vi "Mapping Channel and Image.vi"(9 "Channel Info Index In":u16, 10 "Channel Name":string, 11 "Operation":T2(ring)) -> (1 "Channel Info Index Out":u16, 2 "Channel Info":T1)   [LabVIEW 2021, in "myRIOMetaDataObj.lvclass"]
uses:
  myRIOMetaDataObj.lvclass
  ChannelInfo.ctl
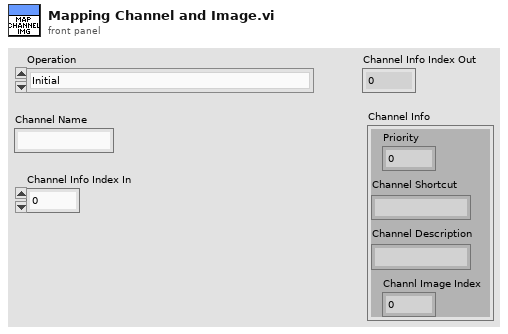
[diagram p1: front panel]
types:
  T1 = typedef "myRIOMetaDataObj.lvclass/ChannelInfo.ctl" = cluster{"Priority":u16, "Channel Shortcut":string, "Channel Description":string, "Channl Image Index":u16}
  T2 = enum16{"Initial", "Get Channel Info Index by Name", "Get Channel Info by Index", "Get Channel Info by Img Index"}
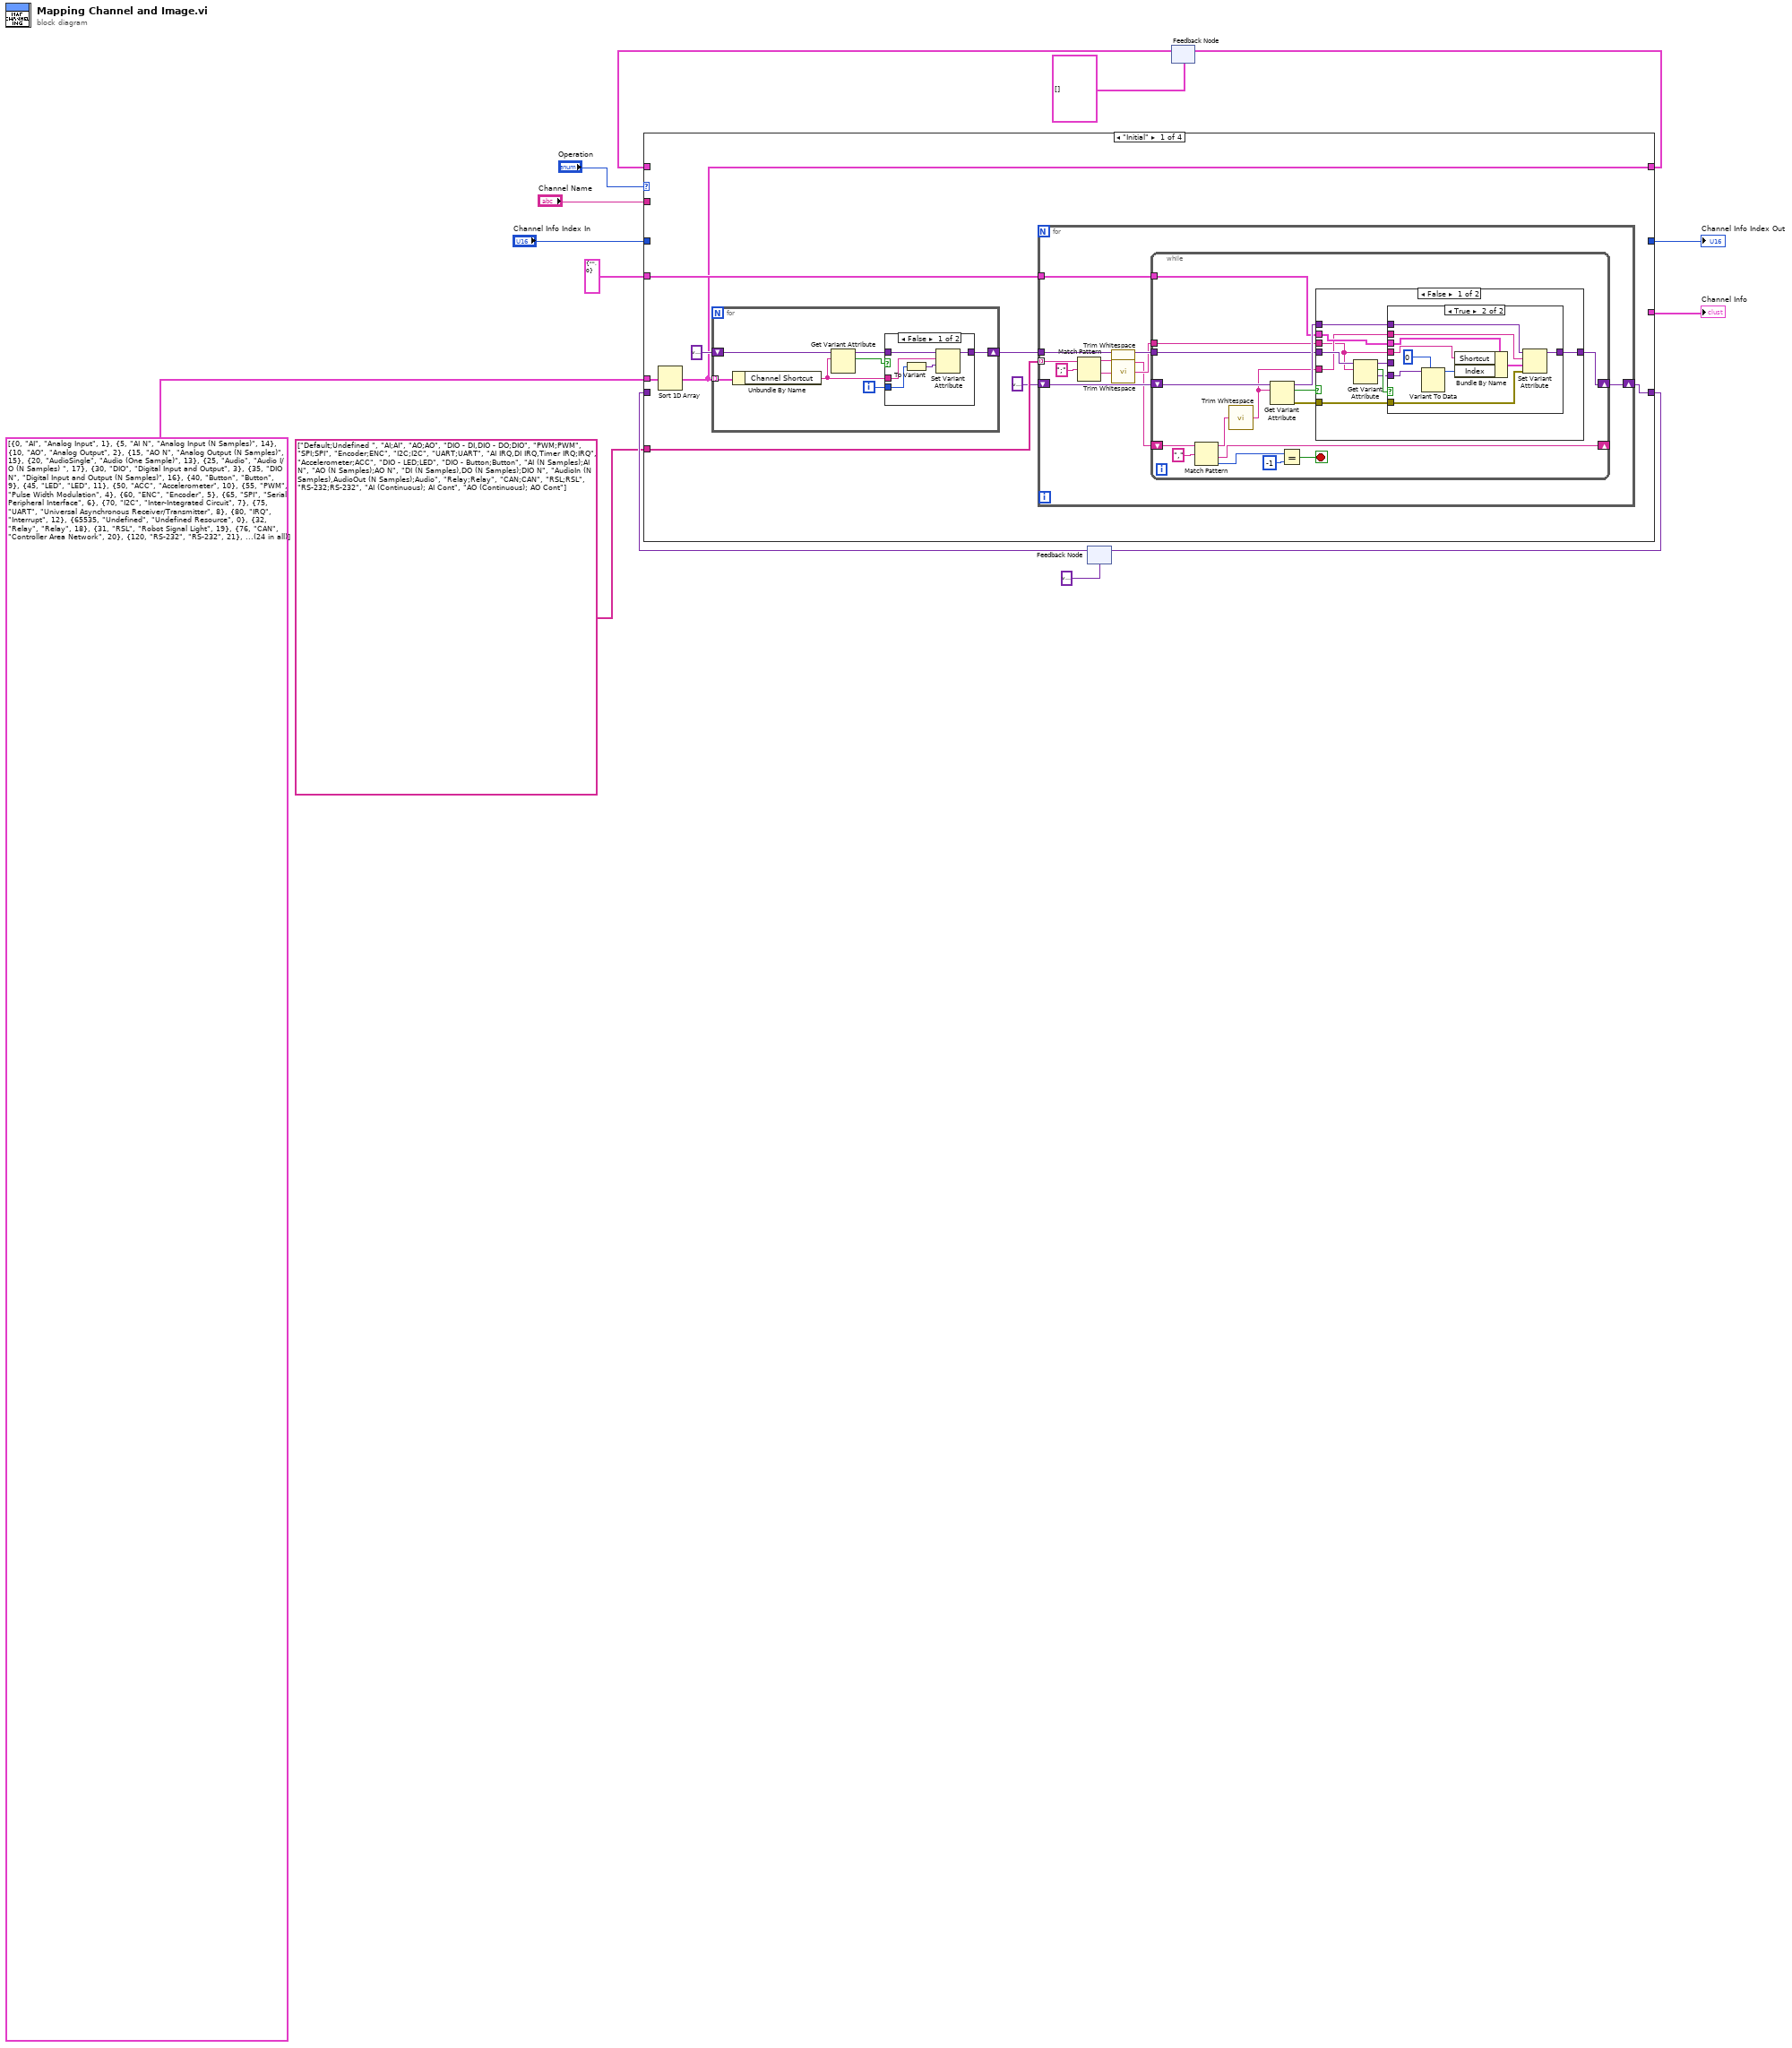
[diagram p0: block diagram]
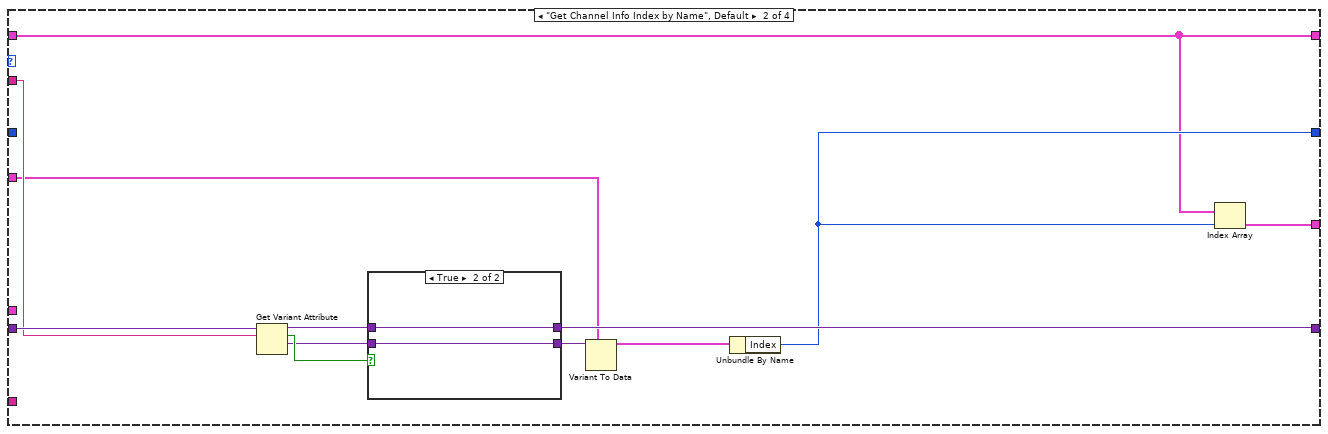
[diagram p5: hidden frame]
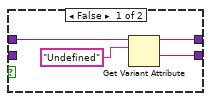
[diagram p6: hidden frame]
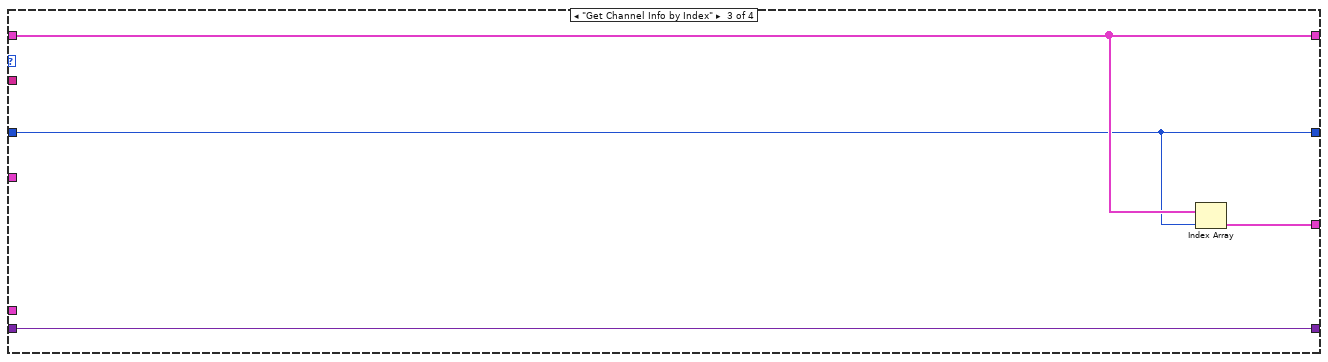
[diagram p7: hidden frame]
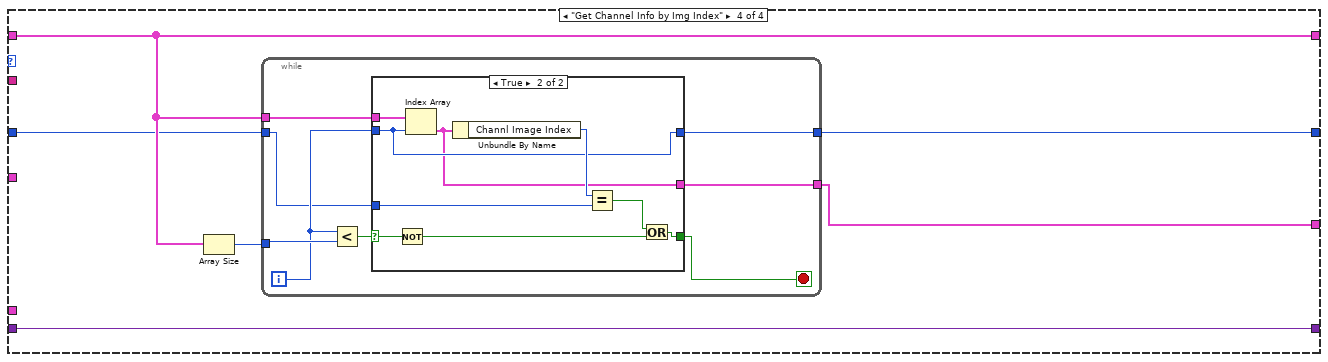
[diagram p8: hidden frame]
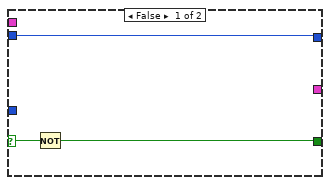
[diagram p9: hidden frame]
diagram:
  n1 = feedback #1(variant ("Channel Info Map in")) -> (w8:variant)
  n2 = feedback #2(T1[] []) -> (w4:T1[])
  n3 = case shown="\"Initial\"" "Operation" {
    tunnel: "Channel Name" -> [_ w94 _ _]
    tunnel: "Channel Info Index In" -> [_ _ w103 w106]
    tunnel: [_ w85 w103 w108] -> w11
    tunnel: T1[] [{"Priority"=0, "Channel Shortcut"="AI", "Channel Description"="Analog Input", "Channl Image Index"=1}, {"Priority"=5, "Channel Shortcut"="AI N", "Channel Description"="Analog Input (N Samples)", "Channl Image Index"=14}, {"Priority"=10, "Channel Shortcut"="AO", "Channel Description"="Analog Output", "Channl Image Index"=2}, {"Priority"=15, "Channel Shortcut"="AO N", "Channel Description"="Analog Output (N Samples)", "Channl Image Index"=15}, {"Priority"=20, "Channel Shortcut"="AudioSingle", "Channel Description"="Audio (One Sample)", "Channl Image Index"=13}, {"Priority"=25, "Channel Shortcut"="Audio", "Channel Description"="Audio I/O (N Samples) ", "Channl Image Index"=17}, {"Priority"=30, "Channel Shortcut"="DIO", "Channel Description"="Digital Input and Output", "Channl Image Index"=3}, {"Priority"=35, "Channel Shortcut"="DIO N", "Channel Description"="Digital Input and Output (N Samples)", "Channl Image Index"=16}, {"Priority"=40, "Channel Shortcut"="Button", "Channel Description"="Button", "Channl Image Index"=9}, {"Priority"=45, "Channel Shortcut"="LED", "Channel Description"="LED", "Channl Image Index"=11}, {"Priority"=50, "Channel Shortcut"="ACC", "Channel Description"="Accelerometer", "Channl Image Index"=10}, {"Priority"=55, "Channel Shortcut"="PWM", "Channel Description"="Pulse Width Modulation", "Channl Image Index"=4}, {"Priority"=60, "Channel Shortcut"="ENC", "Channel Description"="Encoder", "Channl Image Index"=5}, {"Priority"=65, "Channel Shortcut"="SPI", "Channel Description"="Serial Peripheral Interface", "Channl Image Index"=6}, {"Priority"=70, "Channel Shortcut"="I2C", "Channel Description"="Inter-Integrated Circuit", "Channl Image Index"=7}, {"Priority"=75, "Channel Shortcut"="UART", "Channel Description"="Universal Asynchronous Receiver/Transmitter", "Channl Image Index"=8}, {"Priority"=80, "Channel Shortcut"="IRQ", "Channel Description"="Interrupt", "Channl Image Index"=12}, {"Priority"=65535, "Channel Shortcut"="Undefined", "Channel Description"="Undefined Resource", "Channl Image Index"=0}, {"Priority"=32, "Channel Shortcut"="Relay", "Channel Description"="Relay", "Channl Image Index"=18}, {"Priority"=31, "Channel Shortcut"="RSL", "Channel Description"="Robot Signal Light", "Channl Image Index"=19}, {"Priority"=76, "Channel Shortcut"="CAN", "Channel Description"="Controller Area Network", "Channl Image Index"=20}, {"Priority"=120, "Channel Shortcut"="RS-232", "Channel Description"="RS-232", "Channl Image Index"=21}, {"Priority"=6, "Channel Shortcut"="AI Cont", "Channel Description"="Analog Input (Continuous)", "Channl Image Index"=22}, {"Priority"=16, "Channel Shortcut"="AO Cont", "Channel Description"="Analog Output (Continuous)", "Channl Image Index"=23}] -> [w19 _ _ _]
    tunnel: w8 -> [_ w95 w105 w111]
    tunnel: string[] ["Default;Undefined ", "AI;AI", "AO;AO", "DIO - DI,DIO - DO;DIO", "PWM;PWM", "SPI;SPI", "Encoder;ENC", "I2C;I2C", "UART;UART", "AI IRQ,DI IRQ,Timer IRQ;IRQ", "Accelerometer;ACC", "DIO - LED;LED", "DIO - Button;Button", "AI (N Samples);AI N", "AO (N Samples);AO N", "DI (N Samples),DO (N Samples);DIO N", "AudioIn (N Samples),AudioOut (N Samples);Audio", "Relay;Relay", "CAN;CAN", "RSL;RSL", "RS-232;RS-232", "AI (Continuous); AI Cont", "AO (Continuous); AO Cont"] -> [w22 _ _ _]
    tunnel: [w20 w90 w105 w111] -> w6
    tunnel: w4 -> [_ w84 w104 w109]
    tunnel: [w15 w84 w104 w109] -> w1
    tunnel: cluster{"Shortcut":string, "Index":u16} {"Shortcut"="", "Index"=0} ("Shortcut Mapping") -> [w18 w88 _ _]
    tunnel: [_ w86 w102 w107] -> w2
    frame "Initial" {
      n4 = Sort 1D Array(array=w19) -> (sorted array=w15:T1[])
      n5 = for {
        shift-right: [w25] -> w16
        shift-left: variant ("Channel Info Map in") -> [w29]
        tunnel: w15 -> [w28] mode=indexing
        i -> [w23]
        n6 = Unbundle By Name(w28) -> ("Channel Shortcut"=w24:string)
        n7 = Get Variant Attribute(Variant=w29, name=w24) -> (duplicate Variant=w26:variant, found=w27:bool)  [unwired: 2 in, 2 out]
        n8 = case shown="False" w27 {
          tunnel: w26 -> [w34 w35]
          tunnel: [w30 w35] -> w25
          tunnel: w24 -> [w33 _]
          tunnel: w23 -> [w31 _]
          frame False {
            n9 = To Variant(anything=w31) -> (Variant=w32:variant)
            n10 = Set Variant Attribute(Variant=w34, name=w33, value=w32) -> (Variant out=w30:variant)  [unwired: 1 in, 2 out]
          }
          frame True {
          }
        }
      }
      n11 = for {
        tunnel: w22 -> [w45] mode=indexing
        shift-right: [w42] -> w20
        shift-left: variant ("Channel Info Map in") -> [w43]
        tunnel: w18 -> [w41]
        tunnel: w16 -> [w40]
        n12 = Match Pattern(string=w45, regular expression=";" ("search string/char (-)")) -> (before substring=w37:string, after substring=w39:string)  [unwired: 1 in, 2 out]
        n13 = call <vilib>:"Trim Whitespace.vi"("string"=w37) -> ("trimmed string"=w36:string)  [unwired: 1 in]
        n14 = call <vilib>:"Trim Whitespace.vi"("string"=w39) -> ("trimmed string"=w38:string)  [unwired: 1 in]
        n15 = while {
          shift-right: [w46] -> _
          shift-left: w36 -> [w60]
          shift-right: [w52] -> w42
          shift-left: w43 -> [w56]
          tunnel: w38 -> [w50]
          tunnel: w41 -> [w51]
          tunnel: w40 -> [w49]
          stop <- w57 stop-if-true
          n16 = Match Pattern(string=w60, regular expression="," ("search string/char (-)")) -> (before substring=w48:string, after substring=w46:string, offset past match=w59:i32)  [unwired: 1 in, 1 out]
          n17 = call <vilib>:"Trim Whitespace.vi"("string"=w48) -> ("trimmed string"=w47:string)  [unwired: 1 in]
          n18 = Get Variant Attribute(Variant=w56, name=w47) -> (duplicate Variant=w53:variant, found=w55:bool, error out=w54:errorcluster)  [unwired: 2 in, 1 out]
          n19 = Equal?(x=w59, y=-1) -> (x = y?=w57:bool)
          n20 = case shown="False" w55 {
            tunnel: w54 -> [w70 _]
            tunnel: w53 -> [w71 w83]
            tunnel: [w64 w83] -> w52
            tunnel: w47 -> [w67 _]
            tunnel: w51 -> [w69 _]
            tunnel: w50 -> [w62 _]
            tunnel: w49 -> [w68 _]
            frame False {
              n21 = Get Variant Attribute(Variant=w68, name=w62) -> (duplicate Variant=w63:variant, found=w66:bool, value=w65:variant)  [unwired: 2 in, 1 out]
              n22 = case shown="True" w66 {
                tunnel: w71 -> [w72 w82]
                tunnel: w70 -> [_ w81]
                tunnel: w69 -> [_ w80]
                tunnel: w62 -> [_ w79]
                tunnel: w67 -> [_ w78]
                tunnel: w65 -> [_ w77]
                tunnel: [w72 w73] -> w64
                tunnel: w63 -> [_ _]
                frame False {
                  # "Undefined Shortcut"
                }
                frame True {
                  n23 = Variant To Data(type=u16 0 ("Index"), Variant=w77) -> (data=w75:u16)  [unwired: 1 in, 1 out]
                  n24 = Bundle By Name(cluster=w80, "Shortcut"=w79, "Index"=w75) -> (w74:cluster{"Shortcut":string, "Index":u16})
                  n25 = Set Variant Attribute(Variant=w82, name=w78, value=w74, error in=w81) -> (Variant out=w73:variant)  [unwired: 2 out]
                }
              }
            }
            frame True {
              # "Redefined Mapping"
            }
          }
        }
      }
    }
    frame "Get Channel Info Index by Name", Default {
      n26 = Get Variant Attribute(Variant=w95, name=w94) -> (duplicate Variant=w92:variant, found=w93:bool, value=w91:variant)  [unwired: 2 in, 1 out]
      n27 = case shown="True" w93 {
        tunnel: w92 -> [w99 w101]
        tunnel: w91 -> [_ w100]
        tunnel: [w96 w101] -> w90
        tunnel: [w97 w100] -> w89
        frame False {
          n28 = Get Variant Attribute(Variant=w99, name="Undefined") -> (duplicate Variant=w96:variant, value=w97:variant)  [unwired: 2 in, 2 out]
        }
        frame True {
        }
      }
      n29 = Variant To Data(type=w88, Variant=w89) -> (data=w87:cluster{"Shortcut":string, "Index":u16})  [unwired: 1 in, 1 out]
      n30 = Unbundle By Name(w87) -> ("Index"=w85:u16)
      n31 = Index Array(array=w84, index=w85) -> (element=w86:T1)
    }
    frame "Get Channel Info by Index" {
      n32 = Index Array(array=w104, index=w103) -> (element=w102:T1)
    }
    frame "Get Channel Info by Img Index" {
      n33 = Array Size(array=w109) -> (size(s)=w110:i32)
      n34 = while {
        tunnel: w110 -> [w119]
        tunnel: w109 -> [w116]
        tunnel: [w114] -> w108
        tunnel: [w113] -> w107
        tunnel: w106 -> [w112]
        i -> [w115]
        stop <- w117 stop-if-true
        n35 = Less?(x=w115, y=w119) -> (x < y?=w118:bool)
        n36 = case shown="True" w118 {
          selector: w118 -> [w121 w125]
          tunnel: [w120 w129] -> w117
          tunnel: w116 -> [_ w131]
          tunnel: w115 -> [w122 w127]
          tunnel: [w122 w127] -> w114
          tunnel: [_ w126] -> w113
          tunnel: w112 -> [_ w123]
          frame False {
            n37 = Not(x=w121) -> (.not. x?=w120:bool)
          }
          frame True {
            n38 = Not(x=w125) -> (.not. x?=w124:bool)
            n39 = Index Array(array=w131, index=w127) -> (element=w126:T1)
            n40 = Unbundle By Name(w126) -> ("Channl Image Index"=w130:u16)
            n41 = Equal?(x=w130, y=w123) -> (x = y?=w128:bool)
            n42 = Or(x=w128, y=w124) -> (x .or. y?=w129:bool)
          }
        }
      }
    }
  }
  "Channel Info Index Out" <- w11
  "Channel Info" <- w2
  n43 = feedback-in #1(w6) -> ()
  n44 = feedback-in #2(w1) -> ()
